vi "CallMultiGrid.vi"(8 "error in (no error)":errorcluster, 11 "vi path":path) -> (0 "error out":errorcluster)   [LabVIEW 2014]
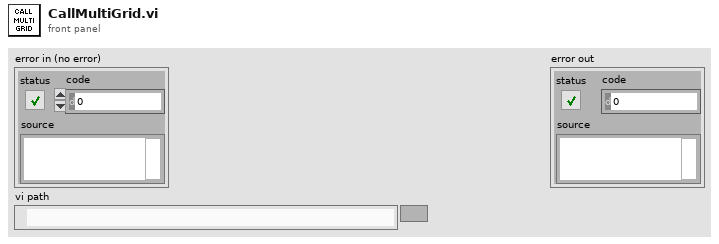
[diagram p1: front panel]
types:
  T1 = enum32{"Invalid", "Standard", "Closed", "Hidden", "Minimized", "Maximized"}
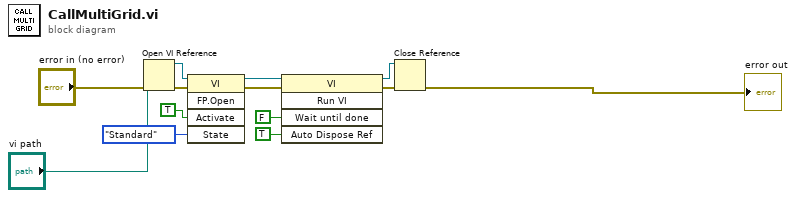
[diagram p0: block diagram]
diagram:
  n1 = Open VI Reference(vi path="vi path", error in (no error)="error in (no error)") -> (vi reference=w12:refnum<vi>, error out=w10:errorcluster)  [unwired: 4 in]
  n2 = invoke class="VI" method="FP.Open"(reference=w12, error in=w10, "Activate"=TRUE ("Activate?"), "State"=T1."Standard") -> (reference out=w11:refnum<vi>, error out=w9:errorcluster)  [unwired: 1 in, 3 out]
  n3 = invoke class="VI" method="Run VI"(reference=w11, error in=w9, "Wait until done"=FALSE ("Wait Until Done"), "Auto Dispose Ref"=TRUE ("Auto Dispose Reference")) -> (reference out=w7:refnum<vi>, error out=w6:errorcluster)  [unwired: 1 in, 3 out]
  n4 = Close Reference(reference=w7, error in (no error)=w6) -> (error out=→"error out":errorcluster)
